vi "Write Value Type Code.vi"(8 "error in (no error)":errorcluster, 10 "type code":T1, 11 "NT Base in":refnum<class "NT Base.lvclass">) -> (0 "error out":errorcluster, 3 "NT Base out":refnum<class "NT Base.lvclass">)   [LabVIEW 2020, in "PV Access.lvlib" / "PV Data.lvlib" / "NT Base.lvclass"]
uses:
  NT Base.lvclass
  NT Base.lvclass/NT Base.ctl
  Type Code.ctl
  PV Data.lvlib
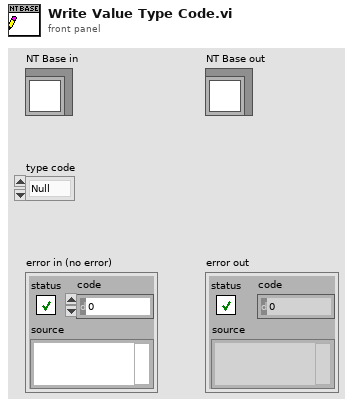
[diagram p1: front panel]
types:
  T1 = typedef "PV Access.lvlib/PV Data.lvlib/Type Code.ctl" = enum8{"Null", "Bool", "BoolA", "Int8", "Int8A", "Int16", "Int16A", "Int32", "Int32A", "Int64", "Int64A", "UInt8", "UInt8A", "UInt16", "UInt16A", "UInt32", "UInt32A", "UInt64", "UInt64A", "Float32", "Float32A", "Float64", "Float64A", "String", "StringA", "Struct", "StructA", "Union", "UnionA", "Any", "AnyA"}
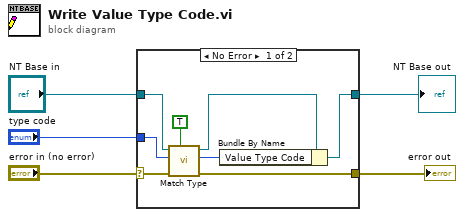
[diagram p0: block diagram]
diagram:
  n1 = case shown="No Error" "error in (no error)" {
    selector: "error in (no error)" -> [w11 w14]
    tunnel: [w10 w14] -> w4
    tunnel: [w13 w15] -> w2
    tunnel: "NT Base in" -> [w7 w15]
    tunnel: "type code" -> [w9 _]
    frame No Error {
      n2 = call-dynamic "Match Type.vi"("raise for mismatch?"=TRUE, "error in (no error)"=w11, "type code"=w9, "NT Base in"=w7) -> ("error out"=w10:errorcluster, "type code out"=w8:T1, "NT Base out"=w6:refnum<class "NT Base.lvclass">)  [unwired: 4 in, 1 out]
      n3 = Bundle By Name(cluster=w6, "Value Type Code"=w8) -> (w13:refnum<class "NT Base.lvclass">)
    }
    frame Error {
    }
  }
  "error out" <- w4
  "NT Base out" <- w2
